vi "SetRobotPosition.vi"(2 "Parameter String":string, 3 "Reinit":bool) -> (0 "Error Out":errorcluster, 1 "Increment":bool)   [LabVIEW 2019]
uses:
  sensors.vi
  CheckForErrorsFloat.vi
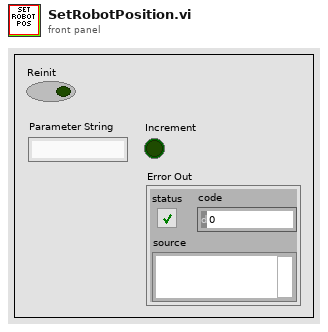
[diagram p1: front panel]
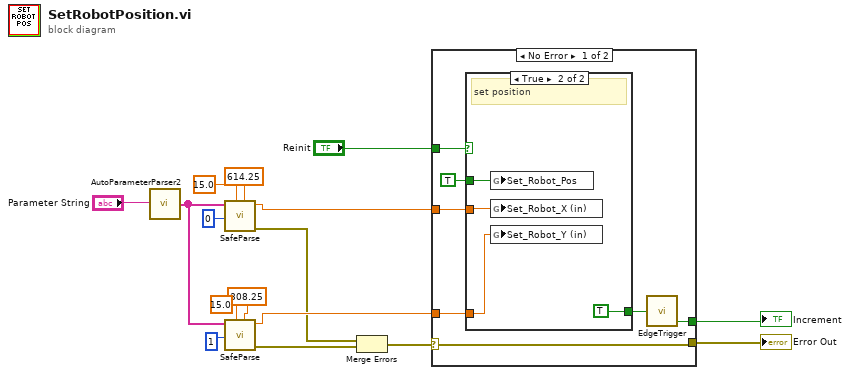
[diagram p0: block diagram]
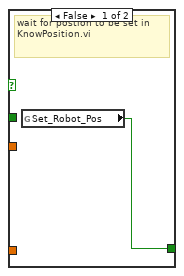
[diagram p2: hidden frame]
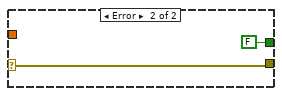
[diagram p3: hidden frame]
diagram:
  n1 = call "AutoParameterParser2.vi"("Parameter String"="Parameter String") -> ("Parsed Parameters"=w7:string[])
  n2 = call-poly "SafeParse.vi"("Maximum"=614.25, "Minimum"=15.0, "Parameter Index"=0, "Parameters"=w7) -> ("Error"=w1:errorcluster, "Output"=w3:dbl)  [unwired: 6 in]
  n3 = call-poly "SafeParse.vi"("Maximum"=308.25, "Minimum"=15.0, "Parameter Index"=1, "Parameters"=w7) -> ("Error"=w4:errorcluster, "Output"=w2:dbl)  [unwired: 6 in]
  n4 = Merge Errors(w1, w4) -> (w5:errorcluster)
  n5 = case shown="No Error" w5 {
    selector: w5 -> [w18 w30]
    tunnel: "Reinit" -> [w23 _]
    tunnel: w3 -> [w22 _]
    tunnel: [w19 FALSE ("Falling Edge Trigger")] -> w15
    tunnel: [w18 w30] -> w14
    tunnel: w2 -> [w17 _]
    frame No Error {
      n6 = case shown="True" w23 {
        tunnel: w22 -> [_ w28]
        tunnel: [w24 TRUE ("Falling Edge Trigger")] -> w20
        tunnel: TRUE -> [_ w26]
        tunnel: w17 -> [_ w25]
        frame False {
          # "wait for postion to be set in KnowPosition.vi"
          n7 = global read "sensors.vi" "Set_Robot_Pos"() -> (w24:bool)
        }
        frame True {
          # "set position"
          n8 = global write "sensors.vi" "Set_Robot_Pos"(w26) -> ()
          n9 = global write "sensors.vi" "Set_Robot_X (in)"(w28) -> ()
          n10 = global write "sensors.vi" "Set_Robot_Y (in)"(w25) -> ()
        }
      }
      n11 = call "EdgeTrigger.vi"("Input Signal"=w20) -> ("Falling Edge Trigger"=w19:bool)  [unwired: 2 out]
    }
    frame Error {
    }
  }
  "Increment" <- w15
  "Error Out" <- w14
